vi "Calibration_Save_2.0.vi"(0 "Img1":T3, 5 "Img2":T3, 7 "Data":T1={"Camera 1"={"Camera1"="", "Cam 1"=FALSE, "CAM1 Model"=enum."a2A5328-15ucBAS", "Cam1 ID"=0}, "Camera 2"={"Camera2"="", "Cam 2"=FALSE, "CAM2 Model"=enum."a2A5328-15ucBAS", "Cam2 ID"=0}, "Image"={"Camera1_Img"=refnum, "Camera2_Img"=refnum, "Img1_Orig_Disp"=refnum, "Img2_Orig_Disp"=refnum, "Img1_Orig_RGB"=refnum, "Img2_Orig_RGB"=refnum, "Blue_Plane_Extract"=refnum, "Subtracted_Plane"=refnum, "Img1_Binary"=refnum, "Img2_Binary"=refnum, "Crop_Mask"=refnum, "Img1_Save"=refnum, "Img2_Save"=refnum, "Img1_Cali_Full"=refnum, "Img2_Cali_Full"=refnum, "Img1_Cali_Detect"=refnum, "Img2_Cali_Detect"=refnum}, "Ques"={"Cam 1 queue"=refnum, "Cam 2 queue"=refnum, "Cam 1 - save queue"=refnum, "Cam 2 - save queue"=refnum, "Image Process Queue Size"=500, "Image Save Queue Size"=500, "Overload threshold"=500, "Max large object threshold"=0}, "Arduino SRS"={"Pinch-valve"="", "Actuator"=FALSE, "Arduino Uno"="", "Valve state"=enum."Open"}, "Pump"={"Port"="", "Connection"=FALSE, "Flush Size"=0, "Command"="", "Pump Size"=enum."None", "Pump"="", "Ready"=FALSE}, "Camera settings"={"Detection settings"={"Sample size threshold"=500, "Detection Region %"=30.0, "Timeout Sample"=200}, "Lens/camera settings"={"Aperture"=enum."Item 0", "Legacy Cam Attributes"=FALSE, "Max Framerate"=100, "Exposure Time"=1000.0, "Framerate"=15}, "Crop settings"={"Cam1"={"Rectangle 1"={"Left"=0, "Top"=0, "Right"=0, "Bottom"=0, "Rotation"=0.0}, "Camera Orientation 1"="", "Pixel to mm 1"=0.0}, "Cam2"={"Rectangle 2"={"Left"=0, "Top"=0, "Right"=0, "Bottom"=0, "Rotation"=0.0}, "Camera Orientation 2"="", "Pixel to mm 2"=0.0}}}, "Arduino ISS"={"Mega F3"="", "Phase3"=FALSE, "Barcode"="", "Sorting sys."=FALSE, "Initial size"=0.0, "Size Interval"=0.0, "Mun. of containers"=0.0, "Container nr."=0.0, "Arduino Mega"=""}, "Img_Capt"=FALSE, "Empty_Refill"=FALSE, "I don't think is in use"={"Light intensity"=100}, "Extended setup"={"Location"="Station", "Latitude"="Station", "Longitude"="Station", "Determiner"="Station", "Sex"="Station", "Station"="", "Collection date"=""}, "Main interface"={"Sample Name"="Test Sample", "Operator"="JFR", "Species Name"="", "Other Notes"=""}, "Tap1"=0, "SystemVersion"=0, "System Serial"="", "Exit"=FALSE, "Kuvette Full"=FALSE, "Core JKI"={"Current VI Reference"=refnum, "Close Panel on Exit?"=FALSE}, "Calibration"={"Calibration 1"=path "C:/Users/au540322/Desktop/IHS_Project/images/Debris/Debris_0/Debris_0_2019_06_01-23-32-49-686.PNG", "Calibration 2"=path "C:/Users/au540322/Desktop/IHS_Project/images/Debris/Debris_0/Debris_0_2019_06_01-23-32-49-686.PNG", "Detect 1"=path "C:/Users/au540322/Desktop/IHS_Project/images/Debris/Debris_0/Debris_0_2019_06_01-23-32-49-686.PNG", "Detect 2"=path "C:/Users/au540322/Desktop/IHS_Project/images/Debris/Debris_0/Debris_0_2019_06_01-23-32-49-686.PNG"}, "Auto Flush"=FALSE, "Status History"="", "Timestamp Start"=""} {"SystemVersion" items=["Standard", "XL"]; "Tap1" items=["Session Data", "Extended Setup", "Buffer", "Camera", "Dispenser", "Stats", "Connections"]; "I don't think is in use"."Light intensity" scale=0.0..100.0; "Camera settings"."Crop settings"."Cam2"."Rectangle 2"."Rotation" format="%.2f"; "Camera settings"."Crop settings"."Cam2"."Rectangle 2"."Left" scale=0.0..1024.0; "Camera settings"."Crop settings"."Cam2"."Rectangle 2"."Right" scale=0.0..1024.0; "Camera settings"."Crop settings"."Cam1"."Rectangle 1"."Rotation" format="%.2f"; "Camera settings"."Crop settings"."Cam1"."Rectangle 1"."Left" scale=0.0..1024.0; "Camera settings"."Crop settings"."Cam1"."Rectangle 1"."Right" scale=0.0..1024.0; "Camera settings"."Lens/camera settings"."Framerate" min=1; "Camera settings"."Lens/camera settings"."Max Framerate" min=1; "Camera settings"."Detection settings"."Sample size threshold" min=1; "Pump"."Flush Size" min=0 max=6000 step=100; "Ques"."Overload threshold" min=1; "Ques"."Image Save Queue Size" min=1; "Ques"."Image Process Queue Size" min=1}, 9 "Dtct":bool, 11 "Crop?":bool) -> (4 "Cal1":path, 6 "Cal2":path, 8 "Data 2":T1={"Camera 1"={"Camera1"="", "Cam 1"=FALSE, "CAM1 Model"=enum."a2A5328-15ucBAS", "Cam1 ID"=0}, "Camera 2"={"Camera2"="", "Cam 2"=FALSE, "CAM2 Model"=enum."a2A5328-15ucBAS", "Cam2 ID"=0}, "Image"={"Camera1_Img"=refnum, "Camera2_Img"=refnum, "Img1_Orig_Disp"=refnum, "Img2_Orig_Disp"=refnum, "Img1_Orig_RGB"=refnum, "Img2_Orig_RGB"=refnum, "Blue_Plane_Extract"=refnum, "Subtracted_Plane"=refnum, "Img1_Binary"=refnum, "Img2_Binary"=refnum, "Crop_Mask"=refnum, "Img1_Save"=refnum, "Img2_Save"=refnum, "Img1_Cali_Full"=refnum, "Img2_Cali_Full"=refnum, "Img1_Cali_Detect"=refnum, "Img2_Cali_Detect"=refnum}, "Ques"={"Cam 1 queue"=refnum, "Cam 2 queue"=refnum, "Cam 1 - save queue"=refnum, "Cam 2 - save queue"=refnum, "Image Process Queue Size"=500, "Image Save Queue Size"=500, "Overload threshold"=500, "Max large object threshold"=0}, "Arduino SRS"={"Pinch-valve"="", "Actuator"=FALSE, "Arduino Uno"="", "Valve state"=enum."Open"}, "Pump"={"Port"="", "Connection"=FALSE, "Flush Size"=0, "Command"="", "Pump Size"=enum."None", "Pump"="", "Ready"=FALSE}, "Camera settings"={"Detection settings"={"Sample size threshold"=500, "Detection Region %"=30.0, "Timeout Sample"=200}, "Lens/camera settings"={"Aperture"=enum."Item 0", "Legacy Cam Attributes"=FALSE, "Max Framerate"=100, "Exposure Time"=1000.0, "Framerate"=15}, "Crop settings"={"Cam1"={"Rectangle 1"={"Left"=0, "Top"=0, "Right"=0, "Bottom"=0, "Rotation"=0.0}, "Camera Orientation 1"="", "Pixel to mm 1"=0.0}, "Cam2"={"Rectangle 2"={"Left"=0, "Top"=0, "Right"=0, "Bottom"=0, "Rotation"=0.0}, "Camera Orientation 2"="", "Pixel to mm 2"=0.0}}}, "Arduino ISS"={"Mega F3"="", "Phase3"=FALSE, "Barcode"="", "Sorting sys."=FALSE, "Initial size"=0.0, "Size Interval"=0.0, "Mun. of containers"=0.0, "Container nr."=0.0, "Arduino Mega"=""}, "Img_Capt"=FALSE, "Empty_Refill"=FALSE, "I don't think is in use"={"Light intensity"=100}, "Extended setup"={"Location"="Station", "Latitude"="Station", "Longitude"="Station", "Determiner"="Station", "Sex"="Station", "Station"="", "Collection date"=""}, "Main interface"={"Sample Name"="Test Sample", "Operator"="JFR", "Species Name"="", "Other Notes"=""}, "Tap1"=0, "SystemVersion"=0, "System Serial"="", "Exit"=FALSE, "Kuvette Full"=FALSE, "Core JKI"={"Current VI Reference"=refnum, "Close Panel on Exit?"=FALSE}, "Calibration"={"Calibration 1"=path "C:/Users/au540322/Desktop/IHS_Project/images/Debris/Debris_0/Debris_0_2019_06_01-23-32-49-686.PNG", "Calibration 2"=path "C:/Users/au540322/Desktop/IHS_Project/images/Debris/Debris_0/Debris_0_2019_06_01-23-32-49-686.PNG", "Detect 1"=path "C:/Users/au540322/Desktop/IHS_Project/images/Debris/Debris_0/Debris_0_2019_06_01-23-32-49-686.PNG", "Detect 2"=path "C:/Users/au540322/Desktop/IHS_Project/images/Debris/Debris_0/Debris_0_2019_06_01-23-32-49-686.PNG"}, "Auto Flush"=FALSE, "Status History"="", "Timestamp Start"=""} {"SystemVersion" items=["Standard", "XL"]; "Tap1" items=["Session Data", "Extended Setup", "Buffer", "Camera", "Dispenser", "Stats", "Connections"]; "I don't think is in use"."Light intensity" scale=0.0..100.0; "Camera settings"."Crop settings"."Cam2"."Rectangle 2"."Rotation" format="%.2f"; "Camera settings"."Crop settings"."Cam2"."Rectangle 2"."Left" scale=0.0..1024.0; "Camera settings"."Crop settings"."Cam2"."Rectangle 2"."Right" scale=0.0..1024.0; "Camera settings"."Crop settings"."Cam1"."Rectangle 1"."Rotation" format="%.2f"; "Camera settings"."Crop settings"."Cam1"."Rectangle 1"."Left" scale=0.0..1024.0; "Camera settings"."Crop settings"."Cam1"."Rectangle 1"."Right" scale=0.0..1024.0; "Camera settings"."Lens/camera settings"."Framerate" min=1; "Camera settings"."Lens/camera settings"."Max Framerate" min=1; "Camera settings"."Detection settings"."Sample size threshold" min=1; "Pump"."Flush Size" min=0 max=6000 step=100; "Ques"."Overload threshold" min=1; "Ques"."Image Save Queue Size" min=1; "Ques"."Image Process Queue Size" min=1}, 10 "Img1 out":T3, 15 "Img2 out":T3)   [LabVIEW 2024]
uses:
  <vilib>/vision/Image Controls.llb/IMAQ Image.ctl
  controls/Data_JKI.ctl
  <vilib>/userDefined/High Color/IMAQdx.ctl
panel:
  out "error out 2":errorcluster
  out "error out":errorcluster
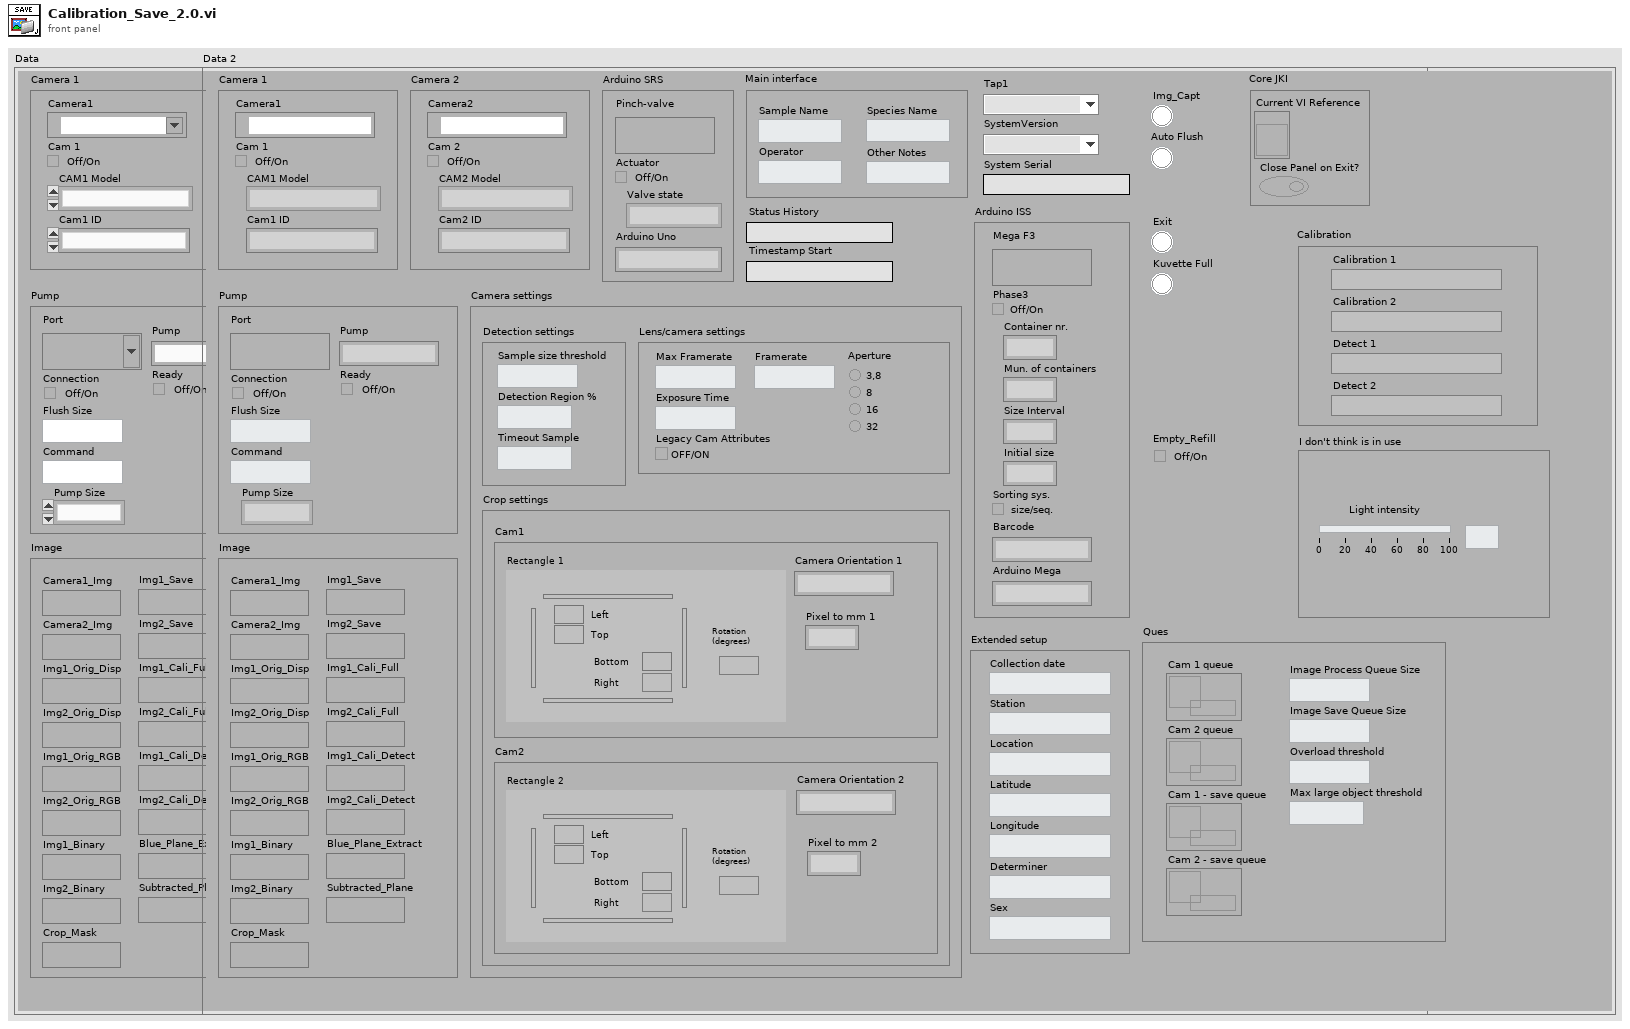
[diagram p1: front panel]
types:
  T1 = typedef "Data_JKI.ctl" = cluster{"Camera 1":cluster{"Camera1":T2, "Cam 1":bool, "CAM1 Model":enum16{"a2A5328-15ucBAS", "acA1920-155uc"}, "Cam1 ID":i32}, "Camera 2":cluster{"Camera2":T2, "Cam 2":bool, "CAM2 Model":enum16{"a2A5328-15ucBAS", "acA1920-155uc"}, "Cam2 ID":i32}, "Image":cluster{"Camera1_Img":T3, "Camera2_Img":T3, "Img1_Orig_Disp":T3, "Img2_Orig_Disp":T3, "Img1_Orig_RGB":T3, "Img2_Orig_RGB":T3, "Blue_Plane_Extract":T3, "Subtracted_Plane":T3, "Img1_Binary":T3, "Img2_Binary":T3, "Crop_Mask":T3, "Img1_Save":T3, "Img2_Save":T3, "Img1_Cali_Full":T3, "Img2_Cali_Full":T3, "Img1_Cali_Detect":T3, "Img2_Cali_Detect":T3}, "Ques":cluster{"Cam 1 queue":refnum<queue>, "Cam 2 queue":refnum<queue>, "Cam 1 - save queue":refnum<queue>, "Cam 2 - save queue":refnum<queue>, "Image Process Queue Size":i32, "Image Save Queue Size":i32, "Overload threshold":i32, "Max large object threshold":i32}, "Arduino SRS":cluster{"Pinch-valve":refnum<visa-resource-name>, "Actuator":bool, "Arduino Uno":string, "Valve state":enum16{"Standby", "Close", "Open"}}, "Pump":cluster{"Port":refnum<visa-resource-name>, "Connection":bool, "Flush Size":i32, "Command":string, "Pump Size":enum16{"None", "Small", "Large"}, "Pump":string, "Ready":bool}, "Camera settings":cluster{"Detection settings":cluster{"Sample size threshold":i32, "Detection Region %":dbl, "Timeout Sample":i32}, "Lens/camera settings":cluster{"Aperture":enum32{"Item 0", "Item 1", "Item 2", "Item 3"}, "Legacy Cam Attributes":bool, "Max Framerate":i32, "Exposure Time":dbl, "Framerate":i32}, "Crop settings":cluster{"Cam1":cluster{"Rectangle 1":T4, "Camera Orientation 1":string, "Pixel to mm 1":dbl}, "Cam2":cluster{"Rectangle 2":T4, "Camera Orientation 2":string, "Pixel to mm 2":dbl}}}, "Arduino ISS":cluster{"Mega F3":refnum<visa-resource-name>, "Phase3":bool, "Barcode":string, "Sorting sys.":bool, "Initial size":dbl, "Size Interval":dbl, "Mun. of containers":dbl, "Container nr.":dbl, "Arduino Mega":string}, "Img_Capt":bool, "Empty_Refill":bool, "I don't think is in use":cluster{"Light intensity":i32}, "Extended setup":cluster{"Location":string, "Latitude":string, "Longitude":string, "Determiner":string, "Sex":string, "Station":string, "Collection date":string}, "Main interface":cluster{"Sample Name":string, "Operator":string, "Species Name":string, "Other Notes":string}, "Tap1":u16, "SystemVersion":u16, "System Serial":string, "Exit":bool, "Kuvette Full":bool, "Core JKI":cluster{"Current VI Reference":refnum<vi>, "Close Panel on Exit?":bool}, "Calibration":cluster{"Calibration 1":path, "Calibration 2":path, "Detect 1":path, "Detect 2":path}, "Auto Flush":bool, "Status History":string, "Timestamp Start":string}
  T2 = typedef "IMAQdx.ctl" = refnum<k21>
  T3 = typedef "IMAQ Image.ctl" = refnum<image>
  T4 = typedef "IMAQ Rectangle" = cluster{"Left":i32, "Top":i32, "Right":i32, "Bottom":i32, "Rotation":dbl}
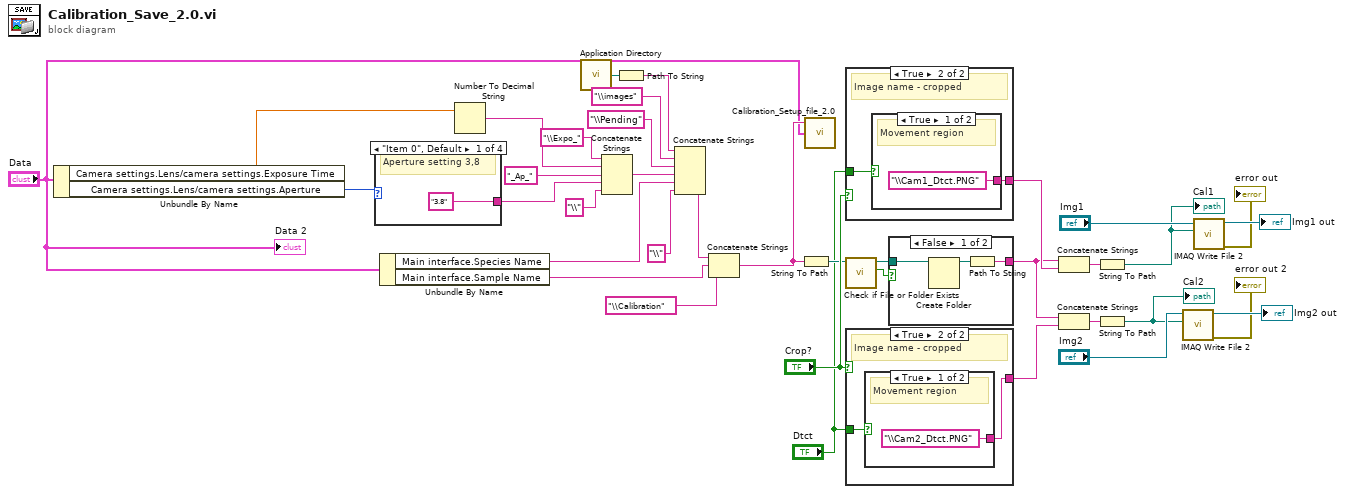
[diagram p0: block diagram]
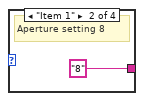
[diagram p2: hidden frame]
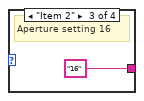
[diagram p3: hidden frame]
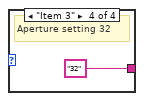
[diagram p4: hidden frame]
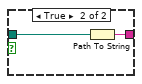
[diagram p5: hidden frame]
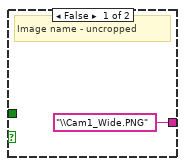
[diagram p6: hidden frame]
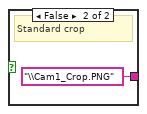
[diagram p7: hidden frame]
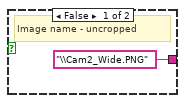
[diagram p8: hidden frame]
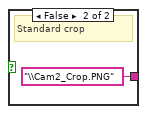
[diagram p9: hidden frame]
diagram:
  n1 = Unbundle By Name("Data") -> ("Camera settings.Lens/camera settings.Exposure Time"=w24:dbl, "Camera settings.Lens/camera settings.Aperture"=w21:enum32{"Item 0", "Item 1", "Item 2", "Item 3"})
  n2 = case shown="\"Item 0\", Default" w21 {
    tunnel: ["3.8" "8" "16" "32"] -> w19
    frame "Item 0", Default {
      # "Aperture setting 3,8"
    }
    frame "Item 1" {
      # "Aperture setting 8"
    }
    frame "Item 2" {
      # "Aperture setting 16"
    }
    frame "Item 3" {
      # "Aperture setting 32"
    }
  }
  n3 = Unbundle By Name("Data") -> ("Main interface.Species Name"=w28:string, "Main interface.Sample Name"=w26:string)
  n4 = Number To Decimal String(number=w24) -> (decimal integer string=w20:string)  [unwired: 1 in]
  n5 = call <vilib>:"Application Directory.vi"() -> ("Application Directory"=w29:path)
  n6 = Concatenate Strings("\\Expo_" ("string"), w20, "_Ap_" ("string"), w19, "\\" ("string")) -> (w17:string)
  n7 = Path To String(path=w29) -> (string=w5:string)
  n8 = Concatenate Strings(w5, "\\images" ("string"), "\\Pending" ("string"), w17, w28, "\\" ("string")) -> (w27:string)
  n9 = Concatenate Strings(w27, w26, "\\Calibration" ("string")) -> (w2:string)
  n10 = String To Path(string=w2) -> (path=w32:path)
  n11 = call "Calibration_Setup_file_2.0.vi"("Data"="Data", "Path"=w2) -> ()  [unwired: 2 in]
  n12 = case shown="True" "Crop?" {
    tunnel: ["\\Cam1_Wide.PNG" ("string") w44] -> w36
    tunnel: "Dtct" -> [_ w43]
    frame False {
      # "Image name - uncropped"
    }
    frame True {
      # "Image name - cropped"
      n13 = case shown="True" w43 {
        tunnel: ["\\Cam1_Dtct.PNG" ("string") "\\Cam1_Crop.PNG" ("string")] -> w44
        frame True {
          # "Movement region"
        }
        frame False {
          # "Standard crop"
        }
      }
    }
  }
  n14 = call <vilib>:"Check if File or Folder Exists.vi"("path"=w32) -> ("file or folder exists?"=w34:bool, "dup path"=w33:path)  [unwired: 8 in, 1 out]
  n15 = case shown="True" "Crop?" {
    tunnel: ["\\Cam2_Wide.PNG" ("string") w49] -> w37
    tunnel: "Dtct" -> [_ w48]
    frame False {
      # "Image name - uncropped"
    }
    frame True {
      # "Image name - cropped"
      n16 = case shown="True" w48 {
        tunnel: ["\\Cam2_Dtct.PNG" ("string") "\\Cam2_Crop.PNG" ("string")] -> w49
        frame True {
          # "Movement region"
        }
        frame False {
          # "Standard crop"
        }
      }
    }
  }
  n17 = case shown="False" w34 {
    tunnel: w33 -> [w54 w56]
    tunnel: [w52 w55] -> w31
    frame False {
      n18 = Create Folder(path (use dialog)=w54) -> (created path=w53:path)  [unwired: 2 in, 2 out]
      n19 = Path To String(path=w53) -> (string=w52:string)
    }
    frame True {
      n20 = Path To String(path=w56) -> (string=w55:string)
    }
  }
  n21 = Concatenate Strings(w31, w36) -> (w14:string)
  n22 = Concatenate Strings(w31, w37) -> (w15:string)
  n23 = String To Path(string=w14) -> (path=w11:path)
  "Cal1" <- w11
  n24 = String To Path(string=w15) -> (path=w10:path)
  "Cal2" <- w10
  n25 = call-poly "IMAQ Write File 2"("File Path"=w10, "Image"="Img2") -> ("error out"=→"error out 2":errorcluster, "Image Out (duplicate)"=→"Img2 out":T3)  [unwired: 8 in]
  n26 = call-poly "IMAQ Write File 2"("File Path"=w11, "Image"="Img1") -> ("error out"=→"error out":errorcluster, "Image Out (duplicate)"=→"Img1 out":T3)  [unwired: 8 in]
  "Data 2" <- "Data"
